vi "LoadResource.vi"(8 "error in (no error)":errorcluster, 9 "Module Root":path, 11 "Resource in":T1) -> (0 "error out":errorcluster, 3 "Resource out":T1)   [LabVIEW 2014]
uses:
  Resource.ctl
  Resource Type.ctl
  Sensor Reading.ctl
  <userlib>/_OpenG.lib/file/file.llb/Build Path - Traditional__ogtk.vi
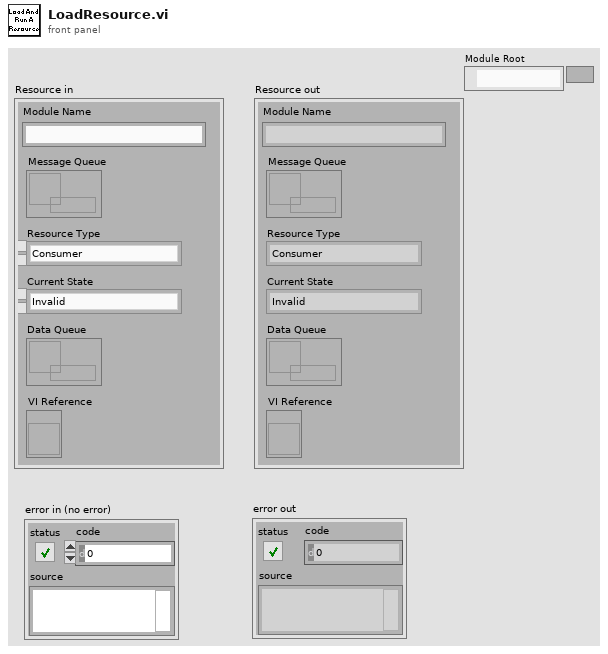
[diagram p1: front panel]
types:
  T1 = typedef "Resource.ctl" = cluster{"Module Name":string, "Message Queue":refnum<queue>, "Resource Type":T2, "Current State":enum16{"Invalid", "InMemory", "Running", "Paused", "Error", ""}, "Data Queue":refnum<queue>, "VI Reference":refnum<vi>}
  T2 = typedef "Resource Type.ctl" = enum16{"Consumer", "Producer", "Observer"}
  T3 = enum16{"Invalid", "InMemory", "Running", "Paused", "Error", ""}
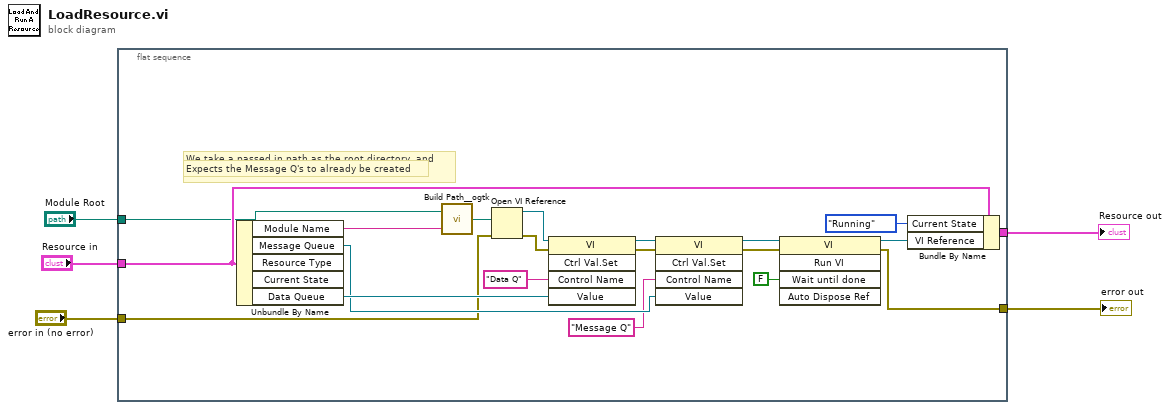
[diagram p0: block diagram]
diagram:
  n1 = flat-sequence {
    tunnel: [w25] -> w5
    tunnel: "Resource in" -> [w22]
    tunnel: "Module Root" -> [w9]
    tunnel: "error in (no error)" -> [w8]
    tunnel: [w7] -> w1
    frame #0 {
      # "We take a passed in path as the root directory, and \nbuild the module path from it."
      # "Expects the Message Q's to already be created"
      n2 = Unbundle By Name(w22) -> ("Module Name"=w6:string, "Message Queue"=w20:refnum<queue>, "Data Queue"=w21:refnum<queue>)  [unwired: 2 out]
      n3 = call-poly <userlib>:"Build Path__ogtk.vi"("name or relative path"=w6, "base path"=w9) -> ("appended path"=w10:path)
      n4 = Open VI Reference(vi path=w10, error in (no error)=w8) -> (vi reference=w11:refnum<vi>, error out=w12:errorcluster)  [unwired: 4 in]
      n5 = invoke class="VI" method="Ctrl Val.Set"(reference=w11, error in=w12, "Control Name"="Data Q", "Value"=w21) -> (reference out=w13:refnum<vi>, error out=w14:errorcluster)  [unwired: 1 in, 3 out]
      n6 = invoke class="VI" method="Ctrl Val.Set"(reference=w13, error in=w14, "Control Name"="Message Q", "Value"=w20) -> (reference out=w17:refnum<vi>, error out=w18:errorcluster)  [unwired: 1 in, 3 out]
      n7 = invoke class="VI" method="Run VI"(reference=w17, error in=w18, "Wait until done"=FALSE ("Wait Until Done")) -> (reference out=w24:refnum<vi>, error out=w7:errorcluster)  [unwired: 2 in, 3 out]
      n8 = Bundle By Name(cluster=w22, "Current State"=T3."Running", "VI Reference"=w24) -> (w25:T1)
    }
  }
  "Resource out" <- w5
  "error out" <- w1
